vi "Load INI Config.vi"(8 "error in":errorcluster, 11 "Config path":path=path "C:/GitHub/Submodule_EOL/Config/INI Config.ini") -> (0 "error out":errorcluster={"status"=TRUE, "code"=7, "source"="NI_LVConfig.lvlib:Load.vi<ERR>\nC:\\Github\\Submodule_Tester\\Config\\INI Config.ini\n\n\n<b>Complete call chain:</b>\r\n     NI_LVConfig.lvlib:Load.vi\r\n     NI_LVConfig.lvlib:Open Config Data.vi\r\n     Load INI Config.vi"})   [LabVIEW 2021]
uses:
  Controls/MUX_Data.ctl
  Controls/DMM_Data.ctl
  Controls/ACIR_Data.ctl
  Controls/HiPOT_Data.ctl
  Controls/DAQ_Data.ctl
  <vilib>/Utility/config.llb/Read Key (String).vi
  <vilib>/Utility/config.llb/NI_LVConfig.lvlib
panel:
  out "data":T1[](array[typedef])
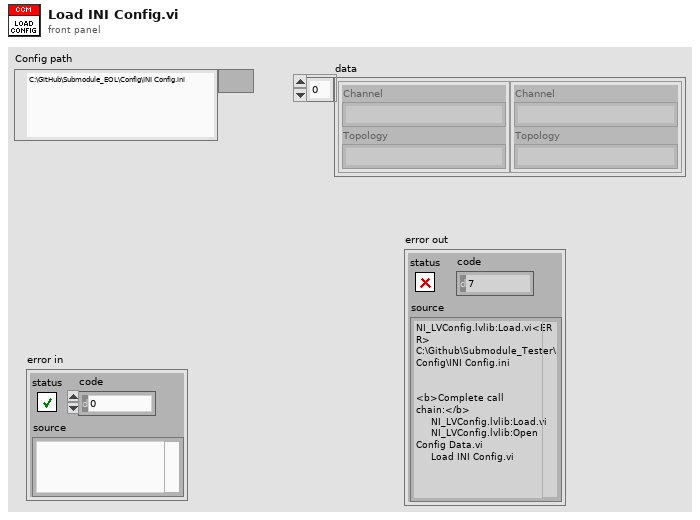
[diagram p1: front panel]
types:
  T1 = typedef "MUX_Data.ctl" = cluster{"Channel":string, "Topology":string}
  T2 = typedef "NI_LVConfig.lvlib/Config Data RefNum.ctl" = refnum<k1>
  T3 = typedef "DMM_Data.ctl" = cluster{"Channel":string, "MUX":string, "Route":string}
  T4 = typedef "ACIR_Data.ctl" = cluster{"Alias":string, "Channel":string}
  T5 = typedef "HiPOT_Data.ctl" = cluster{"Alias":string, "Channel":string}
  T6 = typedef "DAQ_Data.ctl" = cluster{"Alias":string, "DAQ Ch":string}
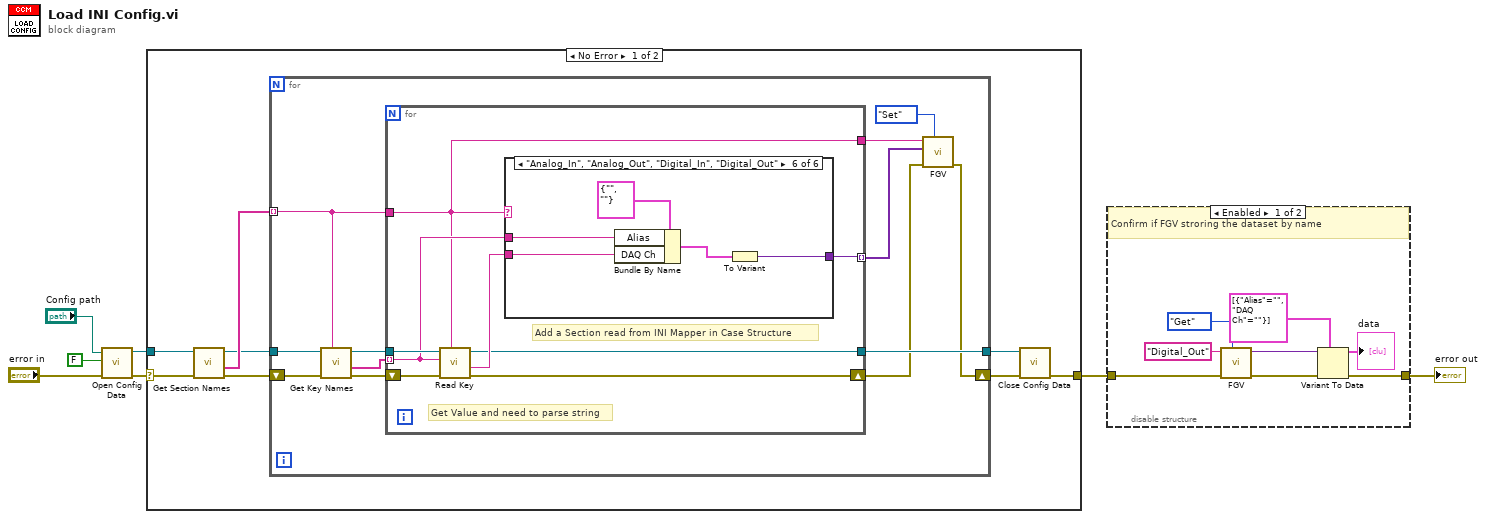
[diagram p0: block diagram]
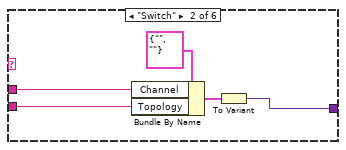
[diagram p3: hidden frame]
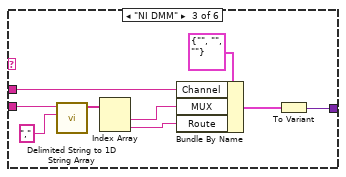
[diagram p4: hidden frame]
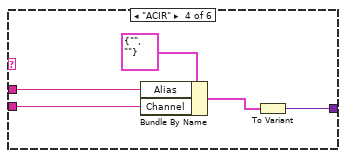
[diagram p5: hidden frame]
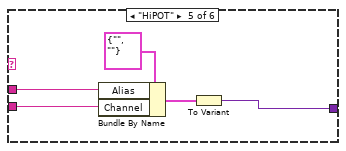
[diagram p6: hidden frame]
diagram:
  n1 = call <vilib>:"Open Config Data.vi"("error in (no error)"="error in", "create file if necessary (T)"=FALSE, "configuration file path"="Config path") -> ("error out"=w5:errorcluster, "refnum"=w6:T2)  [unwired: 6 in, 1 out]
  n2 = case shown="No Error" w5 {
    selector: w5 -> [w15 w65]
    tunnel: [w8 w65] -> w2
    tunnel: w6 -> [w14 _]
    frame No Error {
      n3 = call <vilib>:"Get Section Names.vi"("error in (no error)"=w15, "refnum"=w14) -> ("error out"=w12:errorcluster, "section names"=w13:string[], "refnum out"=w11:T2)  [unwired: 7 in]
      n4 = for {
        tunnel: w13 -> [w24] mode=indexing
        tunnel: w11 -> [w26]
        tunnel: [w25] -> w10
        shift-right: [w17] -> w9
        shift-left: w12 -> [w27]
        n5 = call <vilib>:"Get Key Names.vi"("section"=w24, "error in (no error)"=w27, "refnum"=w26) -> ("error out"=w23:errorcluster, "key names"=w22:string[], "refnum out"=w21:T2)  [unwired: 5 in, 1 out]
        n6 = for {
          tunnel: w22 -> [w32] mode=indexing
          tunnel: w24 -> [w28]
          tunnel: w21 -> [w34]
          tunnel: [w30] -> w25
          tunnel: [w29] -> w19 mode=indexing
          tunnel: [w28] -> w16
          shift-right: [w33] -> w18
          shift-left: w23 -> [w35]
          # "Add a Section read from INI Mapper in Case Structure"
          # "Get Value and need to parse string"
          n7 = call-poly <vilib>:"Read Key.vi"("section"=w28, "error in (no error)"=w35, "key"=w32, "refnum"=w34) -> ("error out"=w33:errorcluster, "value"=w31:string, "refnum out"=w30:T2)  [unwired: 4 in, 1 out]
          n8 = case shown="\"Analog_In\", \"Analog_Out\", \"Digital_In\", \"Digital_Out\"" w28 {
            tunnel: w32 -> [_ w39 w43 w54 w57 w63]
            tunnel: w31 -> [_ w38 w46 w53 w58 w62]
            tunnel: [_ w37 w44 w51 w55 w61] -> w29
            frame Default {
            }
            frame "Switch" {
              n9 = Bundle By Name(cluster=T1 {"Channel"="", "Topology"=""}, "Channel"=w39, "Topology"=w38) -> (w36:T1)
              n10 = To Variant(anything=w36) -> (Variant=w37:variant)
            }
            frame "NI DMM" {
              n11 = call <vilib>:"Delimited String to 1D String Array.vi"("delimiter"=",", "delimited string"=w46) -> ("string array"=w48:string[])  [unwired: 9 in]
              n12 = Index Array(array=w48) -> (element #1=w42:string, element #2=w41:string)  [unwired: 2 in]
              n13 = Bundle By Name(cluster=T3 {"Channel"="", "MUX"="", "Route"=""} ("DAQ Data"), "Channel"=w43, "MUX"=w42, "Route"=w41) -> (w45:T3)
              n14 = To Variant(anything=w45) -> (Variant=w44:variant)
            }
            frame "ACIR" {
              n15 = Bundle By Name(cluster=T4 {"Alias"="", "Channel"=""} ("ACIR Data"), "Alias"=w54, "Channel"=w53) -> (w52:T4)
              n16 = To Variant(anything=w52) -> (Variant=w51:variant)
            }
            frame "HiPOT" {
              n17 = Bundle By Name(cluster=T5 {"Alias"="", "Channel"=""} ("HiPOT Data"), "Alias"=w57, "Channel"=w58) -> (w59:T5)
              n18 = To Variant(anything=w59) -> (Variant=w55:variant)
            }
            frame "Analog_In", "Analog_Out", "Digital_In", "Digital_Out" {
              n19 = Bundle By Name(cluster=T6 {"Alias"="", "DAQ Ch"=""} ("DAQ Data"), "Alias"=w63, "DAQ Ch"=w62) -> (w64:T6)
              n20 = To Variant(anything=w64) -> (Variant=w61:variant)
            }
          }
        }
        n21 = call "FGV.vi"("Method (Get)"=enum16{"Get", "Set"}."Set", "error in"=w18, "Data In"=w19, "Name"=w16) -> ("error out"=w17:errorcluster)  [unwired: 6 in, 1 out]
      }
      n22 = call <vilib>:"Close Config Data.vi"("error in (no error)"=w9, "refnum"=w10) -> ("error out"=w8:errorcluster)  [unwired: 8 in, 1 out]
    }
    frame Error {
    }
  }
  n23 = disable-structure "Diagram Disable Structure" shown="Enabled" {
    disable-tunnel: w2 -> [w73 w74]
    disable-tunnel: [w69 w74] -> w1
    frame Enabled {
      # "Confirm if FGV stroring the dataset by name"
      n24 = call "FGV.vi"("Method (Get)"=enum16{"Get", "Set"}."Get", "error in"=w73, "Name"="Digital_Out") -> ("error out"=w71:errorcluster, "Data out"=w70:variant)  [unwired: 7 in]
      n25 = Variant To Data(error in=w71, type=T6[] [{"Alias"="", "DAQ Ch"=""}], Variant=w70) -> (data=→"data":T6[], error out=w69:errorcluster)
    }
    frame Disabled {
    }
  }
  "error out" <- w1
